vi "openloop.vi"() -> ()   [LabVIEW 2018]
uses:
  <vilib>/Analysis/_algsub.llb/Vector Norm.vi
  <vilib>/Analysis/_algsub.llb/Real Vector Norm.vi
  <vilib>/Analysis/baseanly.llb/Outer Product.vi
  <vilib>/Analysis/baseanly.llb/Real Outer Product.vi
  <vilib>/robotics/Kinematics/Create Lie Group Matrix.vi
  <vilib>/Analysis/baseanly.llb/Real Inverse Matrix.vi
  <vilib>/imath/engines/lvmath2/RunTimeEngine/NodeEndStatement/NIMS_NodeEndStatement_Output.vi
  <instcachedir>/0/NIMS_NodeEndStatement_Output_53EC0D466D134D7ABD903AC30B43404B.lvgen/NIMS_NodeEndStatement_Output_53EC0D466D134D7ABD903AC30B43404B_005.vi
  <instcachedir>/0/NIMS_NodeEndStatement_Output_53EC0D466D134D7ABD903AC30B43404B.lvgen/NIMS_NodeEndStatement_Output_53EC0D466D134D7ABD903AC30B43404B_000.vi
  <instcachedir>/0/NIMS_NodeEndStatement_Output_53EC0D466D134D7ABD903AC30B43404B.lvgen/NIMS_NodeEndStatement_Output_53EC0D466D134D7ABD903AC30B43404B_002.vi
  <vilib>/imath/engines/lvmath2/RunTimeEngine/ErrorHandling/NIMS_Finalize Error.vi
  <vilib>/Analysis/Matrix/Numeric/Conversions/Matrix To Array - RM.vi
  <vilib>/imath/engines/lvmath2/RunTimeEngine/IndexRead/NIMS M(S,S).vi
  <instcachedir>/0/NIMS M(S,S)_AC51E74150A542F7991B9634C66F3096.lvgen/NIMS M(S,S)_AC51E74150A542F7991B9634C66F3096_000.vi
  <vilib>/imath/engines/lvmath2/RunTimeEngine/BuiltInFunctions/abs/NIMS_abs(signed).vi
  <instcachedir>/0/NIMS_abs(signed)_C4FCB8E6058B49B797C7C8D53CA5F6EC.lvgen/NIMS_abs(signed)_C4FCB8E6058B49B797C7C8D53CA5F6EC_000.vi
  <vilib>/imathl/engines/lvmath/Functions/Error Handling/Create Error.vi
  <vilib>/imath/engines/lvmath2/RunTimeEngine/BuiltInFunctions/atan2/NIMS_atan2.vi
  <instcachedir>/0/NIMS_atan2_A91AA4A7D42247EDBE8F76DB99AF04A4.lvgen/NIMS_atan2_A91AA4A7D42247EDBE8F76DB99AF04A4_002.vi
  <vilib>/imath/engines/lvmath2/RunTimeEngine/ErrorHandling/NIMS_Create Error From Enums.vi
  <vilib>/imath/engines/lvmath2/RunTimeEngine/BuiltInFunctions/cos/NIMS_cos(C).vi
  <instcachedir>/0/NIMS_cos(C)_96B8A70E6B8E4D29AD8526A89C8CF3DF.lvgen/NIMS_cos(C)_96B8A70E6B8E4D29AD8526A89C8CF3DF_001.vi
  <instcachedir>/0/NIMS_atan2_A91AA4A7D42247EDBE8F76DB99AF04A4.lvgen/NIMS_atan2_A91AA4A7D42247EDBE8F76DB99AF04A4_001.vi
  <vilib>/imath/engines/lvmath2/RunTimeEngine/IndexRead/NIMS V(S).vi
  <instcachedir>/0/NIMS V(S)_0488751826AF41519A22953C041130DC.lvgen/NIMS V(S)_0488751826AF41519A22953C041130DC_003.vi
  <vilib>/imath/engines/lvmath2/RunTimeEngine/BuiltInFunctions/sin/NIMS_sin(C).vi
  <instcachedir>/0/NIMS_sin(C)_7FE83C8DCD97403BBE687635FA1F837E.lvgen/NIMS_sin(C)_7FE83C8DCD97403BBE687635FA1F837E_001.vi
  <instcachedir>/0/NIMS V(S)_0488751826AF41519A22953C041130DC.lvgen/NIMS V(S)_0488751826AF41519A22953C041130DC_000.vi
  <vilib>/imath/engines/lvmath2/RunTimeEngine/ArithmeticOperatorToken/NIMS_ArithmeticOperator_multmx.vi
  <instcachedir>/0/NIMS_ArithmeticOperator_multmx_622CA76F9646436AB036D42A9A1CE0E6.lvgen/NIMS_ArithmeticOperator_multmx_622CA76F9646436AB036D42A9A1CE0E6_004.vi
  <vilib>/imath/engines/lvmath2/RunTimeEngine/ArithmeticOperatorToken/NIMS_ArithmeticOperator_multmx(M,CV).vi
  <instcachedir>/0/NIMS_ArithmeticOperator_multmx(M,CV)_2F1CD6A2FE4F4213A4AD1C901C2750F5.lvgen/NIMS_ArithmeticOperator_multmx(M,CV)_2F1CD6A2FE4F4213A4AD1C901C2750F5_000.vi
  <vilib>/imath/engines/lvmath2/RunTimeEngine/ArithmeticOperatorToken/NIMS_ArithmeticOperator_multmx(M,CV)-internal.vi
  <instcachedir>/0/NIMS_ArithmeticOperator_multmx(M,CV)-internal_5287250D8D1D4A3E9F77F5DF08D432E0.lvgen/NIMS_ArithmeticOperator_multmx(M,CV)-internal_5287250D8D1D4A3E9F77F5DF08D432E0_004.vi
  <vilib>/imath/engines/lvmath2/RunTimeEngine/ArithmeticOperatorToken/NIMS_ArithmeticOperator_minus.vi
  <instcachedir>/0/NIMS_ArithmeticOperator_minus_C4D0373119CC411691B2E50DF2E09F22.lvgen/NIMS_ArithmeticOperator_minus_C4D0373119CC411691B2E50DF2E09F22_009.vi
  <instcachedir>/0/NIMS_ArithmeticOperator_multmx_622CA76F9646436AB036D42A9A1CE0E6.lvgen/NIMS_ArithmeticOperator_multmx_622CA76F9646436AB036D42A9A1CE0E6_008.vi
  <vilib>/imath/engines/lvmath2/RunTimeEngine/IndexRead/NIMS M(S).vi
  <instcachedir>/0/NIMS M(S)_B826C018497E4940AE96BD27B540B6FB.lvgen/NIMS M(S)_B826C018497E4940AE96BD27B540B6FB_004.vi
  <vilib>/imath/engines/lvmath2/RunTimeEngine/Managers/WorkSpace/UID Generator.vi
  <vilib>/imath/engines/lvmath2/RunTimeEngine/RunTimeType/NIMS_RunTimeType_From StrictType (excl LVString).vi
  <instcachedir>/0/NIMS_RunTimeType_From StrictType (excl LVString)_E7E34A65C99947108168652BAD14964D.lvgen/NIMS_RunTimeType_From StrictType (excl LVString)_E7E34A65C99947108168652BAD14964D_000.vi
  <vilib>/imath/engines/lvmath2/RunTimeEngine/LocalVariableDefStatement/MC_LocalVariableDefStatement_Display.vi
  <instcachedir>/0/NIMS M(S)_B826C018497E4940AE96BD27B540B6FB.lvgen/NIMS M(S)_B826C018497E4940AE96BD27B540B6FB_000.vi
  <vilib>/imath/engines/lvmath2/RunTimeEngine/Managers/SymbolTable/Clear UID.vi
  <vilib>/Analysis/Matrix/Numeric/Multiply/Multiply.vi
  <vilib>/Analysis/Matrix/Numeric/Multiply/Multiply - RM,R.vi
  <vilib>/Analysis/Matrix/Numeric/Multiply/Multiply - R,RM.vi
  <vilib>/Analysis/Matrix/Numeric/Add/Add.vi
  <vilib>/Analysis/Matrix/Numeric/Add/Add - RM,RM.vi
  <instcachedir>/0/NIMS_NodeEndStatement_Output_53EC0D466D134D7ABD903AC30B43404B.lvgen/NIMS_NodeEndStatement_Output_53EC0D466D134D7ABD903AC30B43404B_001.vi
  <instcachedir>/0/NIMS_NodeEndStatement_Output_53EC0D466D134D7ABD903AC30B43404B.lvgen/NIMS_NodeEndStatement_Output_53EC0D466D134D7ABD903AC30B43404B_008.vi
  <vilib>/imath/engines/lvmath2/RunTimeEngine/IndexRead/NIMS M($,S).vi
  <instcachedir>/0/NIMS M($,S)_3E5749BBB62E49528D4765A77F1F6D98.lvgen/NIMS M($,S)_3E5749BBB62E49528D4765A77F1F6D98_000.vi
  <vilib>/imath/engines/lvmath2/RunTimeEngine/RowToken/NIMS_RowToken_SorRV_CV.vi
  <instcachedir>/0/NIMS_RowToken_SorRV_CV_E9A223509C5746E8B9F22970C86A52C1.lvgen/NIMS_RowToken_SorRV_CV_E9A223509C5746E8B9F22970C86A52C1_000.vi
  <vilib>/Analysis/NI_AALBase.lvlib
  <vilib>/gmath/NI_Gmath.lvlib
  <vilib>/Analysis/Matrix/NI_Matrix.lvlib
  <vilib>/robotics/Kinematics/NI_Kinematics.lvlib
  <vilib>/imath/engines/lvmath2/RunTimeEngine/Managers/SymbolTable/NIMS_WorkSpace.lvlib
panel:
  out "Yaw":cluster{"E1_now":dbl[], "t_now":dbl[]}(graph)
  out "Pitch":cluster{"E1_now":dbl[], "t_now":dbl[]}(graph)
  out "Roll":cluster{"E1_now":dbl[], "t_now":dbl[]}(graph)
  in  "MOI(kg*m^2)":dbl[][](array[numeric])
  in  "COG(m)":dbl[](array[numeric])
  in  "Mass (kg)":dbl
  in  "Simulation Time(sec)":dbl
  # "Physical Parameters"
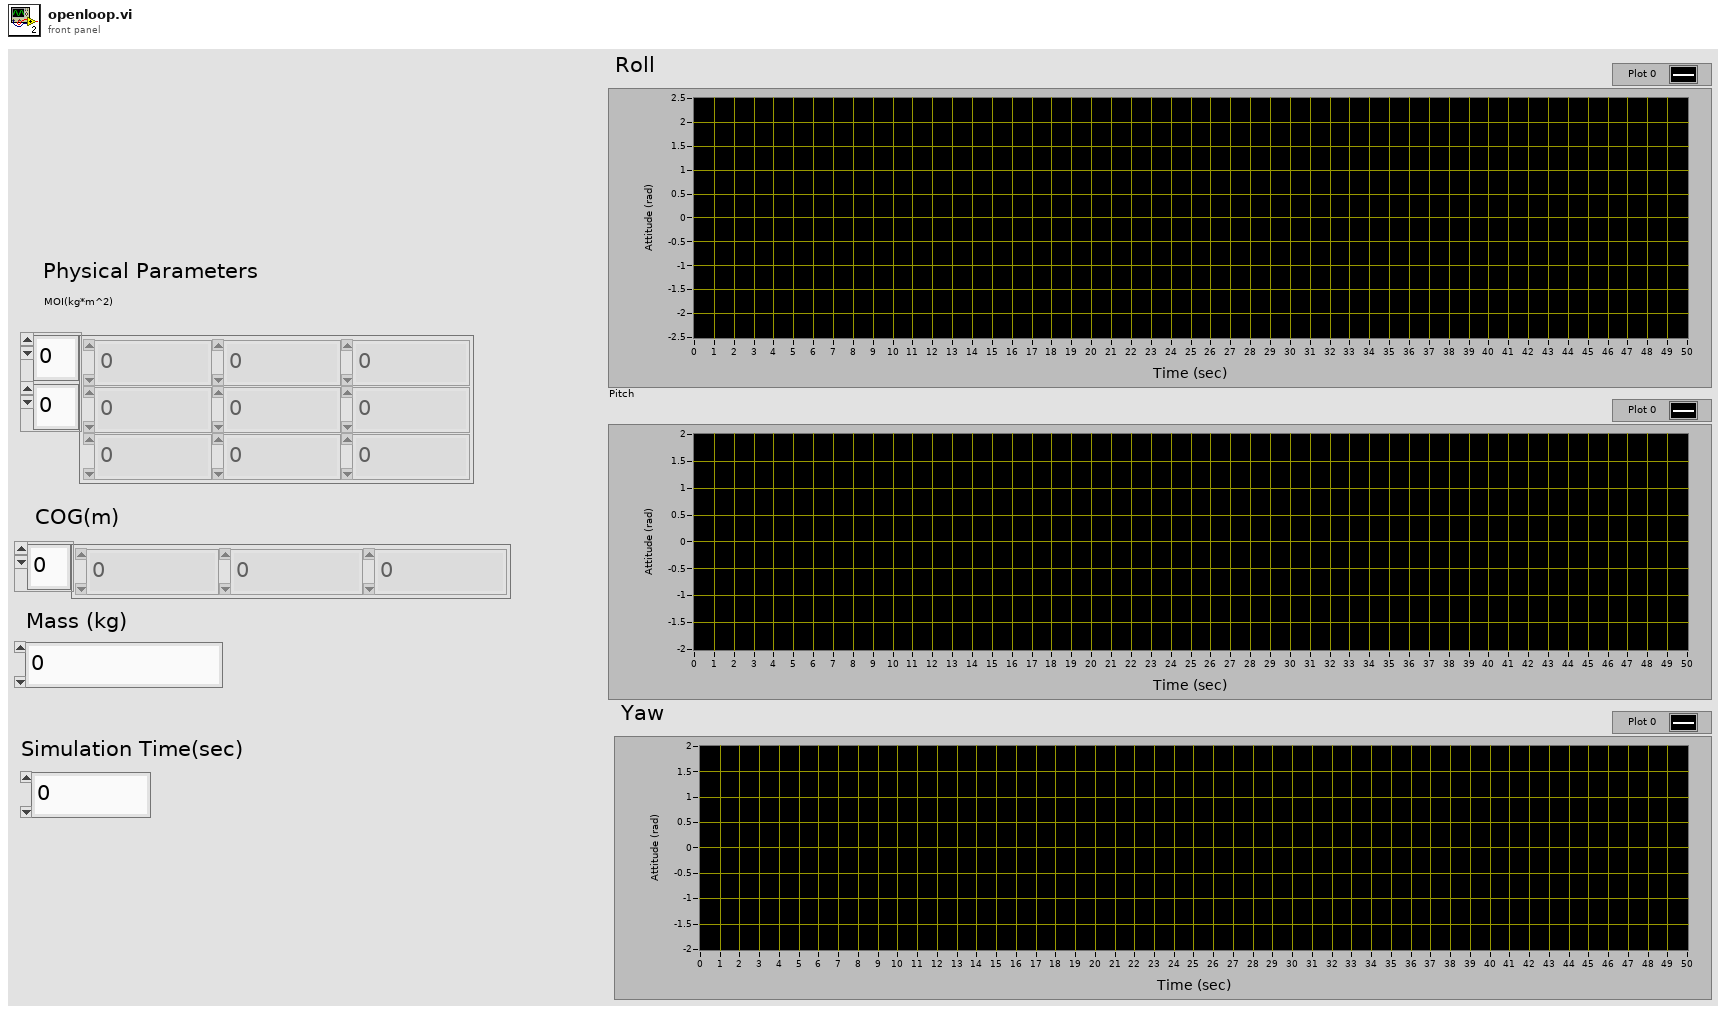
[diagram p1: front panel]
types:
  T1 = cluster{"E1":cdb[], "E2":dbl[], "E3":dbl[], "t":dbl[]}
  T2 = typedef "NI_Matrix.lvlib/RealMatrix.ctl" = dbl[][]
  T3 = typedef "NI_Kinematics.lvlib/Quaternion.ctl" = dbl[]
  T4 = cluster{"E1_now":cdb[], "E2_now":cdb[], "E3_now":dbl[], "t_now":dbl[]}
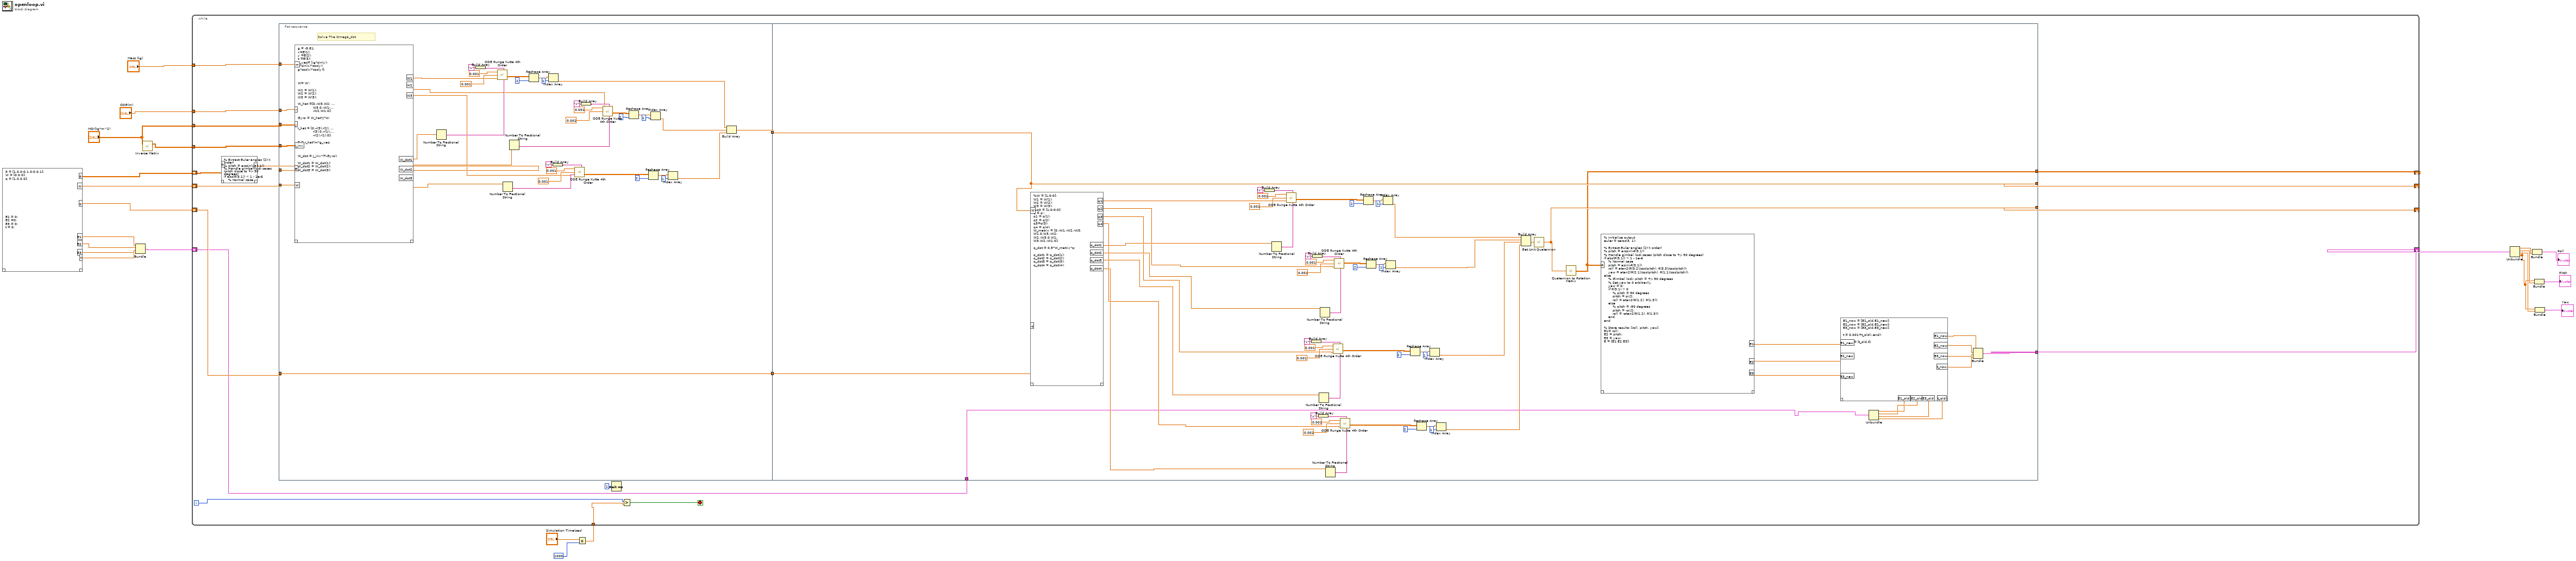
[diagram p0: block diagram]
diagram:
  n1 = mathscript code="R = [1,0,0;0,1,0;0,0,1];\nW = [0,0,0];\nq = [1,0,0,0];\n\n\n\n\n\n\n\n\n\n\nE1 = 0;\nE2 =0;\nE3 = 0;\nt = 0;"() -> ("R"=w16:dbl[][], "W"=w15:dbl[], "q"=w14:dbl[], "E1"=w13:cdb[], "E2"=w12:dbl[], "E3"=w11:dbl[], "t"=w1:dbl[])  [unwired: 1 in, 1 out]
  n2 = Bundle("E1"=w13, "E2"=w12, "E3"=w11, "t"=w1) -> (w10:T1)  [unwired: 1 in]
  n3 = call-poly <vilib>:"Inverse Matrix.vi"("Input Matrix"="MOI(kg*m^2)") -> ("Inverse Matrix"=w18:T2)  [unwired: 1 in, 1 out]
  n4 = Multiply(x="Simulation Time(sec)", y=1000) -> (x*y=w21:dbl)
  n5 = while {
    tunnel: w21 -> [w29]
    tunnel: "Mass (kg)" -> [w38]
    tunnel: "COG(m)" -> [w39]
    tunnel: w18 -> [w41]
    tunnel: "MOI(kg*m^2)" -> [w40]
    shift-right: [w32] -> _
    shift-left: w16 -> [w25]
    shift-right: [w31] -> _
    shift-left: w15 -> [w37]
    shift-right: [w33] -> _
    shift-left: w14 -> [w34]
    shift-right: [w27] -> w9
    shift-left: w10 -> [w28]
    i -> [w24]
    stop <- w30 stop-if-true
    n6 = mathscript code="% Extract Euler angles (ZYX order)\n% pitch = arcsin(-R(3,1))\n% Handle gimbal lock cases (pitch close to +/- 90 degrees)\nif abs(R(3,1)) < 1 - 1e-6\n    % Normal case\n    pitch = asin(-R(3,1));\n    roll = atan2(R(3,2)/cos(pitch), R(3,3)/cos(pitch));\n    yaw = atan2(R(2,1)/cos(pitch), R(1,1)/cos(pitch));\nelse\n    % Gimbal lock: pitch = +/- 90 degrees\n    % Set yaw to 0 arbitrarily\n    yaw = 0;\n    if R(3,1) < 0\n        % pitch = 90 degrees\n        pitch = pi/2;\n        roll = atan2(R(1,2), R(1,3));\n    else\n        % pitch = -90 degrees\n        pitch = -pi/2;\n        roll = -atan2(R(1,2), R(1,3));\n    end\nend\n\n% Store results: [roll, pitch, yaw]\nE1= roll;\nE2 = pitch;\nE3 = yaw;\nE = [E1,E2,E3];"("R"=w25) -> ("E"=w36:cdb[])  [unwired: 1 in, 1 out]
    n7 = flat-sequence {
      tunnel: [w320] -> w35
      tunnel: [w319] -> w26
      tunnel: w36 -> [w362]
      tunnel: w41 -> [w361]
      tunnel: w40 -> [w360]
      tunnel: w39 -> [w359]
      tunnel: w38 -> [w358]
      tunnel: w37 -> [w357]
      tunnel: w34 -> [w320]
      tunnel: w35 -> [w782]
      tunnel: [w781] -> w33
      tunnel: [w779] -> w32
      tunnel: [w780] -> w31
      tunnel: w28 -> [w772]
      tunnel: [w768] -> w27
      tunnel: w26 -> [w780]
      frame #0 {
        # "Solve The Omega_dot"
        n8 = mathscript code="g = -9.81;\nx=E(1);\ny =E(2);\nz =E(3);\ng_vec= [-g*sin(y);\ng*sin(x)*cos(y);\ng*cos(x)*cos(y)];\n\n\n\nW= W';\n\nW1 = W(1);\nW2 = W(2);\nW3 = W(3);\n\nW_hat =[0,-W3,W2; ...\n              W3,0,-W1;...\n              -W2,W1,0];\n\nGyro = W_hat*J*W;\n\n\nr_hat = [0,-r(3),r(2); ...\n              r(3),0,-r(1);...\n              -r(2),r(1),0];\n\nT = r_hat*m*g_vec;\n\n\n\nW_dot = J_inv*(T-Gyro);\n\nW_dot1 = W_dot(1);\nW_dot2 = W_dot(2);\nW_dot3 = W_dot(3);"("E"=w362, "J"=w360, "J_inv"=w361, "r"=w359, "m"=w358, "W"=w357) -> ("W_dot1"=w321:dbl[], "W_dot2"=w322:dbl[], "W_dot3"=w323:dbl[], "W1"=w326:dbl[], "W2"=w325:dbl[], "W3"=w324:dbl[])  [unwired: 1 in, 1 out]
        n9 = Number To Fractional String(number=w321) -> (F-format string=w352:string[])  [unwired: 3 in]
        n10 = Build Array("x") -> (w355:string[])
        n11 = call <vilib>:"ODE Runge Kutta 4th Order.vi"("time end"=0.001, "h (step rate)"=0.001, "X0"=w326, "X (name of variables)"=w355, "F(X,t) (right sides of the ODE\nas functions of X and t)"=w352) -> ("X Values (solution)"=w348:dbl[][])  [unwired: 2 in, 3 out]
        n12 = Number To Fractional String(number=w323) -> (F-format string=w334:string[])  [unwired: 3 in]
        n13 = Number To Fractional String(number=w322) -> (F-format string=w343:string[])  [unwired: 3 in]
        n14 = Reshape Array(w348, 2 ("dimension size")) -> (w350:dbl[])
        n15 = Index Array(array=w350, index=1) -> (element=w329:dbl)
        n16 = Build Array("x") -> (w337:string[])
        n17 = call <vilib>:"ODE Runge Kutta 4th Order.vi"("time end"=0.001, "h (step rate)"=0.001, "X0"=w324, "X (name of variables)"=w337, "F(X,t) (right sides of the ODE\nas functions of X and t)"=w334) -> ("X Values (solution)"=w330:dbl[][])  [unwired: 2 in, 3 out]
        n18 = Build Array("x") -> (w346:string[])
        n19 = call <vilib>:"ODE Runge Kutta 4th Order.vi"("time end"=0.001, "h (step rate)"=0.001, "X0"=w325, "X (name of variables)"=w346, "F(X,t) (right sides of the ODE\nas functions of X and t)"=w343) -> ("X Values (solution)"=w339:dbl[][])  [unwired: 2 in, 3 out]
        n20 = Reshape Array(w339, 2 ("dimension size")) -> (w341:dbl[])
        n21 = Reshape Array(w330, 2 ("dimension size")) -> (w332:dbl[])
        n22 = Index Array(array=w341, index=1) -> (element=w328:dbl)
        n23 = Index Array(array=w332, index=1) -> (element=w327:dbl)
        n24 = Build Array(w329, w328, w327) -> (w319:dbl[])
      }
      frame #1 {
        n25 = mathscript code="%W = [1;0;0];\nW1 = W(1);\nW2 = W(2);\nW3 = W(3);\n%q0 = [1;0;0;0];\nq = q';\nq1 = q(1);\nq2 = q(2)\nq3=q(3);\nq4 = q(4);\nW_matrix = [0,-W1,-W2,-W3;\nW1,0,W3,-W2;\nW2,-W3,0,W1;\nW3,W2,-W1,0];\n\nq_dot = 0.5*W_matrix*q;\n\nq_dot1 = q_dot(1);\nq_dot2 = q_dot(2);\nq_dot3 = q_dot(3);\nq_dot4 = q_dot(4);"("q"=w782, "W"=w780) -> ("q_dot1"=w821:dbl[], "q_dot2"=w810:dbl[], "q_dot3"=w799:dbl[], "q_dot4"=w788:dbl[], "q1"=w822:dbl[], "q2"=w811:dbl[], "q3"=w800:dbl[], "q4"=w789:dbl[])  [unwired: 1 in, 1 out]
        n26 = Build Array("x") -> (w830:string[])
        n27 = Number To Fractional String(number=w821) -> (F-format string=w827:string[])  [unwired: 3 in]
        n28 = call <vilib>:"ODE Runge Kutta 4th Order.vi"("time end"=0.001, "h (step rate)"=0.001, "X0"=w822, "X (name of variables)"=w830, "F(X,t) (right sides of the ODE\nas functions of X and t)"=w827) -> ("X Values (solution)"=w823:dbl[][])  [unwired: 2 in, 3 out]
        n29 = Build Array("x") -> (w808:string[])
        n30 = Build Array("x") -> (w819:string[])
        n31 = Build Array("x") -> (w797:string[])
        n32 = Number To Fractional String(number=w799) -> (F-format string=w805:string[])  [unwired: 3 in]
        n33 = Number To Fractional String(number=w810) -> (F-format string=w816:string[])  [unwired: 3 in]
        n34 = Number To Fractional String(number=w788) -> (F-format string=w794:string[])  [unwired: 3 in]
        n35 = call <vilib>:"ODE Runge Kutta 4th Order.vi"("time end"=0.001, "h (step rate)"=0.001, "X0"=w800, "X (name of variables)"=w808, "F(X,t) (right sides of the ODE\nas functions of X and t)"=w805) -> ("X Values (solution)"=w801:dbl[][])  [unwired: 2 in, 3 out]
        n36 = call <vilib>:"ODE Runge Kutta 4th Order.vi"("time end"=0.001, "h (step rate)"=0.001, "X0"=w811, "X (name of variables)"=w819, "F(X,t) (right sides of the ODE\nas functions of X and t)"=w816) -> ("X Values (solution)"=w812:dbl[][])  [unwired: 2 in, 3 out]
        n37 = call <vilib>:"ODE Runge Kutta 4th Order.vi"("time end"=0.001, "h (step rate)"=0.001, "X0"=w789, "X (name of variables)"=w797, "F(X,t) (right sides of the ODE\nas functions of X and t)"=w794) -> ("X Values (solution)"=w790:dbl[][])  [unwired: 2 in, 3 out]
        n38 = Reshape Array(w823, 2 ("dimension size")) -> (w825:dbl[])
        n39 = Reshape Array(w812, 2 ("dimension size")) -> (w814:dbl[])
        n40 = Index Array(array=w825, index=1) -> (element=w787:dbl)
        n41 = Index Array(array=w814, index=1) -> (element=w786:dbl)
        n42 = Reshape Array(w801, 2 ("dimension size")) -> (w803:dbl[])
        n43 = Reshape Array(w790, 2 ("dimension size")) -> (w792:dbl[])
        n44 = Index Array(array=w803, index=1) -> (element=w785:dbl)
        n45 = Index Array(array=w792, index=1) -> (element=w784:dbl)
        n46 = Build Array(w787, w786, w785, w784) -> (w783:dbl[])
        n47 = call <vilib>:"Get Unit Quaternion.vi"("quaternion"=w783) -> ("unit quaternion"=w781:T3)
        n48 = call <vilib>:"Quaternion to Rotation Matrix.vi"("quaternion"=w781) -> ("rotation matrix"=w779:T2)
        n49 = mathscript code="% Initialize output\neuler = zeros(3, 1);\n\n% Extract Euler angles (ZYX order)\n% pitch = arcsin(-R(3,1))\n% Handle gimbal lock cases (pitch close to +/- 90 degrees)\nif abs(R(3,1)) < 1 - 1e-6\n    % Normal case\n    pitch = asin(-R(3,1));\n    roll = atan2(R(3,2)/cos(pitch), R(3,3)/cos(pitch));\n    yaw = atan2(R(2,1)/cos(pitch), R(1,1)/cos(pitch));\nelse\n    % Gimbal lock: pitch = +/- 90 degrees\n    % Set yaw to 0 arbitrarily\n    yaw = 0;\n    if R(3,1) < 0\n        % pitch = 90 degrees\n        pitch = pi/2;\n        roll = atan2(R(1,2), R(1,3));\n    else\n        % pitch = -90 degrees\n        pitch = -pi/2;\n        roll = -atan2(R(1,2), R(1,3));\n    end\nend\n\n% Store results: [roll, pitch, yaw]\nE1= roll;\nE2 = pitch;\nE3 = yaw;\nE = [E1,E2,E3];"("R"=w779) -> ("E1"=w778:dbl, "E2"=w777:cdb, "E3"=w776:dbl)  [unwired: 1 in, 1 out]
        n50 = Unbundle(w772) -> ("E1_now"=w775:cdb[], "E2_now"=w774:cdb[], "E3_now"=w773:dbl[], "t_now"=w767:dbl[])
        n51 = mathscript code="E1_now = [E1_old,E1_new];\nE2_now = [E2_old,E2_new];\nE3_now = [E3_old,E3_new];\n\nt = 0.001+t_old(:,end);\n\nt_now = [t_old,t];"("E1_new"=w778, "E2_new"=w777, "E3_new"=w776, "E1_old"=w775, "E2_old"=w774, "E3_old"=w773, "t_old"=w767) -> ("E1_now"=w771:cdb[], "E2_now"=w770:cdb[], "E3_now"=w769:dbl[], "t_now"=w766:dbl[])  [unwired: 1 in, 1 out]
        n52 = Bundle("E1_now"=w771, "E2_now"=w770, "E3_now"=w769, "t_now"=w766) -> (w768:T4)  [unwired: 1 in]
      }
    }
    n53 = Wait (ms)(milliseconds to wait=u32 1) -> ()  [unwired: 1 out]
    n54 = Greater?(x=w24, y=w29) -> (0:w30:bool)
  }
  n55 = Unbundle(w9) -> ("E1_now"=w8:cdb[], "E2_now"=w7:cdb[], "E3_now"=w2:dbl[], "t_now"=w6:dbl[])
  n56 = Bundle("t_now"=w6, "E1_now"=w8) -> (→"Roll":cluster{"t_now":dbl[], "E1_now":cdb[]})  [unwired: 1 in]
  n57 = Bundle("t_now"=w6, "E2_now"=w7) -> (→"Pitch":cluster{"t_now":dbl[], "E2_now":cdb[]})  [unwired: 1 in]
  n58 = Bundle("t_now"=w6, "E3_now"=w2) -> (→"Yaw":cluster{"t_now":dbl[], "E3_now":dbl[]})  [unwired: 1 in]
